vi "Create_Object.vi"(8 "error in (no error)":errorcluster, 9 "Terminal Map in":map{string, T1}(c390), 10 "owner refnum":variant, 11 "Class Specifier Constant in":refnum<class "Class Specifier Constant.lvclass">) -> (0 "error out":errorcluster, 1 "Terminal Map Out":map{string, T1}(c390), 3 "Class Specifier Constant out":refnum<class "Class Specifier Constant.lvclass">)   [LabVIEW 2025, in "Class Specifier Constant.lvclass"]
uses:
  Class Specifier Constant.lvclass
  C:/Users/mrjak/Documents/GitHub/LVGPT/LabVIEW/VIs/Classes/Node/Node.lvclass
  Controls/Terminal.ctl
  Node.lvclass/Node.ctl
  Constant.lvclass
  Node.lvclass
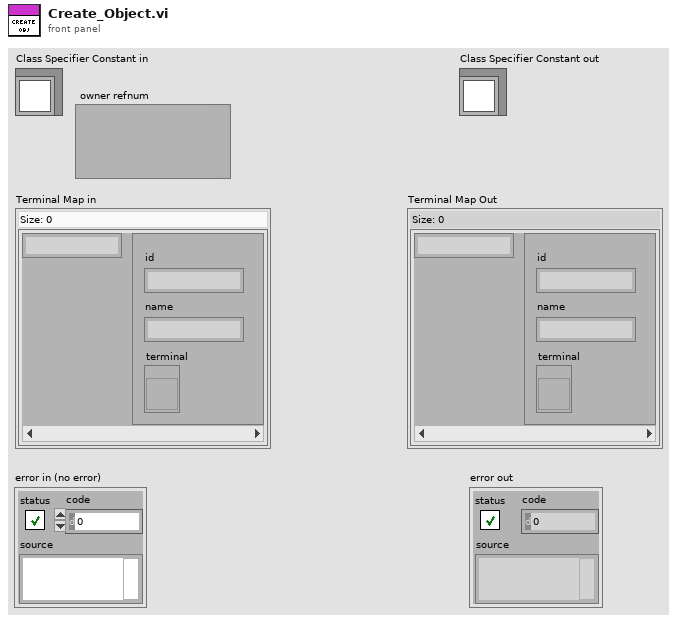
[diagram p1: front panel]
types:
  T1 = typedef "Terminal.ctl" = cluster{"id":string, "name":string, "terminal":refnum<vi>}
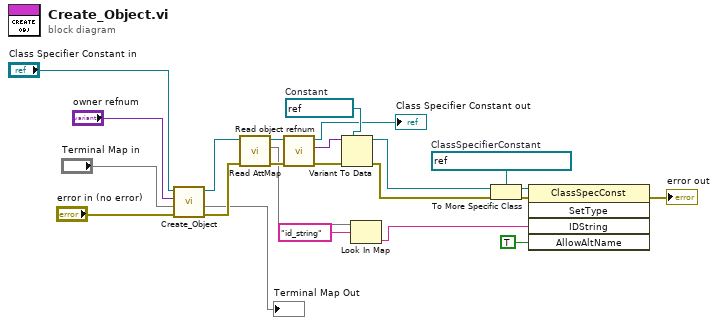
[diagram p0: block diagram]
diagram:
  w7 = refnum<vi> refnum  # ClassSpecifierConstant
  w11 = refnum<vi> refnum  # Constant
  n1 = call-parent "Create_Object.vi"("error in (no error)"="error in (no error)", "Terminal Map in"="Terminal Map in", "owner refnum"="owner refnum", "Constant in"="Class Specifier Constant in") -> ("error out"=w15:errorcluster, "Terminal Map Out"=→"Terminal Map Out":map{string, T1}, "Constant out"=w16:refnum<class "Class Specifier Constant.lvclass">)  [unwired: 5 in]
  n2 = call "Read AttMap.vi"("error in (no error)"=w15, "Node in"=w16) -> ("error out"=w14:errorcluster, "AttMap"=w5:map{string, string}, "Node out"=w13:refnum<class "Class Specifier Constant.lvclass">)  [unwired: 7 in]
  n3 = call-dynamic "Read object refnum.vi"("error in (no error)"=w14, "Node in"=w13) -> ("error out"=w12:errorcluster, "object refnum"=w10:variant, "Node out"=→"Class Specifier Constant out":refnum<class "Class Specifier Constant.lvclass">)  [unwired: 7 in]
  n4 = Variant To Data(error in=w12, type=w11, Variant=w10) -> (data=w9:refnum<vi>, error out=w8:errorcluster)
  n5 = Look In Map(map=w5, key="id_string") -> (value=w4:string)  [unwired: 1 in, 1 out]
  n6 = To More Specific Class(target class=w7, reference=w9) -> (specific class reference=w17:refnum<vi>)  [unwired: 1 in, 1 out]
  n7 = invoke class="ClassSpecConst" method="SetType"(reference=w17, error in=w8, "IDString"=w4, "AllowAltName"=TRUE ("Allow Alternate Name? (F)")) -> (error out=→"error out":errorcluster)  [unwired: 1 in, 4 out]
